vi "torque with filtering trial.vi"() -> ()   [LabVIEW 2018]
panel:
  out "Waveform Graph 2":u32[](graph)
  out "Waveform Graph":sgl[][](graph)
  in  "nominal angle (degrees)":dbl=4.0 format="%#_13g"
  in  "angle error (degrees)":dbl=4.0 format="%#_13g"
  in  "speed (Hz)":i32=666
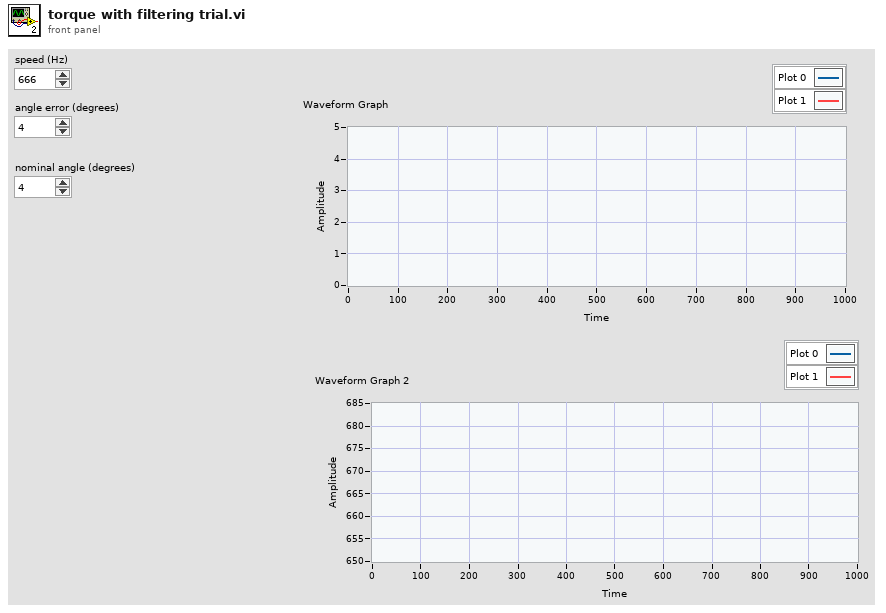
[diagram p1: front panel]
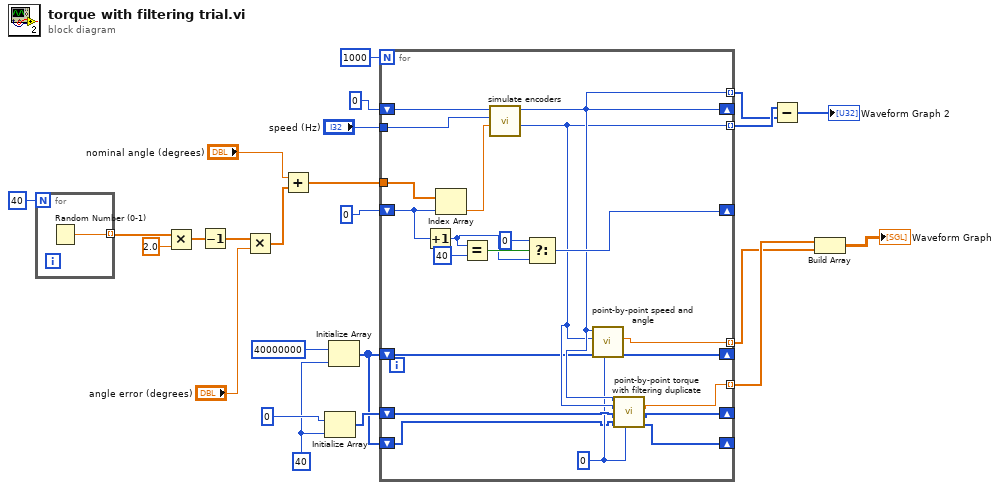
[diagram p0: block diagram]
diagram:
  w8 = 40 ("dimension size")
  n1 = for {
    N: 40 -> [_]
    tunnel: [w25] -> w21 mode=indexing
    n2 = Random Number (0-1)() -> (number: 0 to 1=w25:dbl)
  }
  n3 = Multiply(x=w21, y=2.0 ("Angle (degrees)")) -> (x*y=w19:dbl[])
  n4 = Decrement(x=w19) -> (x-1=w18:dbl[])
  n5 = Multiply(x=w18, y="angle error (degrees)") -> (x*y=w16:dbl[])
  n6 = Add(x="nominal angle (degrees)", y=w16) -> (x+y=w14:dbl[])
  n7 = Initialize Array(0, w8) -> (w7:i32[])
  n8 = Initialize Array(u32 40000000, w8) -> (w3:u32[])
  n9 = for {
    N: 1000 -> [_]
    shift-right: [w34] -> _
    shift-left: u32 0 ("previous tick") -> [w46]
    tunnel: "speed (Hz)" -> [w45]
    tunnel: w14 -> [w44]
    shift-right: [w37] -> _
    shift-left: u32 0 ("previous tick") -> [w42]
    tunnel: [w33] -> w5 mode=indexing
    tunnel: [w34] -> w4 mode=indexing
    shift-right: [w36] -> _
    shift-left: w3 -> [w31]
    tunnel: [w35] -> w1 mode=indexing
    shift-right: [w30] -> _
    shift-left: w7 -> [w32]
    tunnel: [w29] -> w2 mode=indexing
    shift-right: [w26] -> _
    shift-left: w3 -> [w27]
    w28 = u32 0 ("encoders offset")
    n10 = Increment(x=w42) -> (x+1=w39:u32)
    n11 = Index Array(array=w44, index=w42) -> (element=w43:dbl)
    n12 = Equal?(x=w39, y=u32 40) -> (x = y?=w40:bool)
    n13 = call "simulate encoders.vi"("Angle (degrees)"=w43, "speed (Hz)"=w45, "previous tick"=w46) -> ("angle pulse"=w33:u32, "speed pulse"=w34:u32)  [unwired: 7 in]
    n14 = Select(t=u32 0, s=w40, f=w39) -> (s? t:f=w37:u32)
    n15 = call "point-by-point speed and angle.vi"("encoders offset"=w28, "speed history in"=w31, "angle pulse"=w33, "speed pulse"=w34) -> ("speed history out"=w36:u32[], "calculated angle (degrees)"=w35:sgl)  [unwired: 4 in, 2 out]
    n16 = call "point-by-point torque with filtering duplicate.vi"("encoders offset"=w28, "speed history in"=w27, "torque history"=w32, "angle pulse"=w33, "speed pulse"=w34) -> ("speed history out"=w26:u32[], "torque history out"=w30:i32[], "calculated angle (degrees)"=w29:sgl)  [unwired: 2 in, 2 out]
  }
  n17 = Subtract(x=w5, y=w4) -> (x-y=→"Waveform Graph 2":u32[])
  n18 = Build Array(w2, w1) -> (→"Waveform Graph":sgl[][])
